vi "CabecalhoValvulaUnitariaV1.vi"(0 "Output File":path, 1 "Delta t":dbl=1.0, 2 "DAQ Rate":i32=5, 3 "SP CAME Frequency":dbl) -> (4 "data file":string="Data File:    created on Friday, December 03, 1999  at  4:41:37 PM\n\nWARNING: No tampering with this data please.\n\nTomasz W. Wysokinski   Cryofuel Systems Group © 1997/99.\n\n\n Abs. Time \t Run Time\tHCL-VLT\t HeatPipe \t GM-1 \tunused\t SHLD-1\t GM-2\t HCL-bottom\t M-1\t M-2\t SHLD-2\t Hall-P\t Magnet\r")   [LabVIEW 2019]
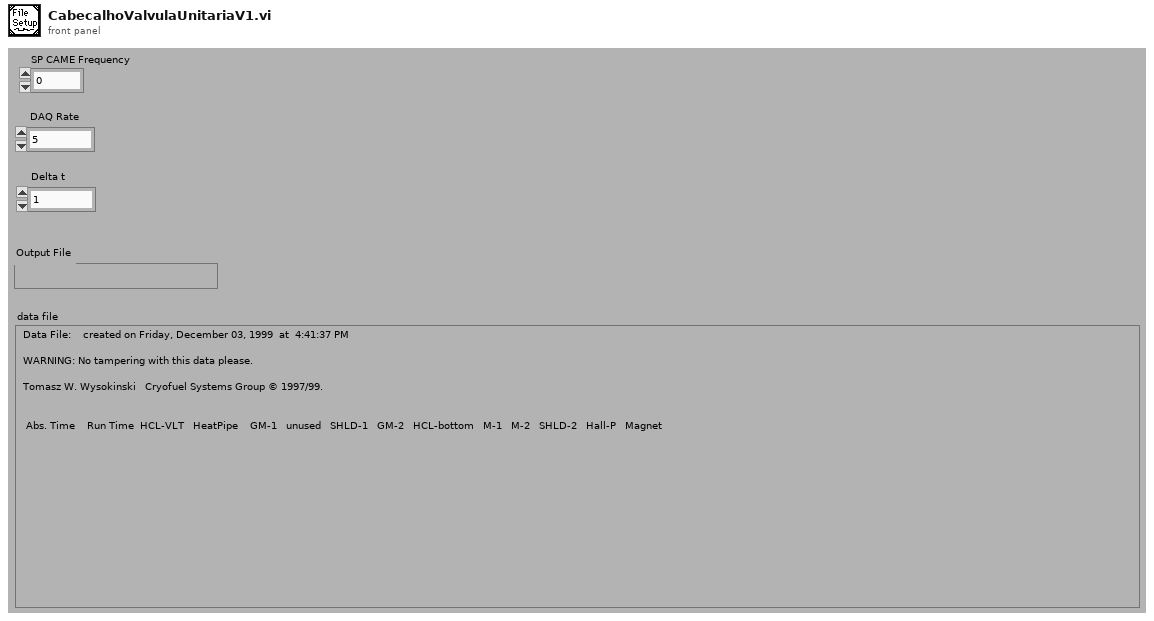
[diagram p1: front panel]
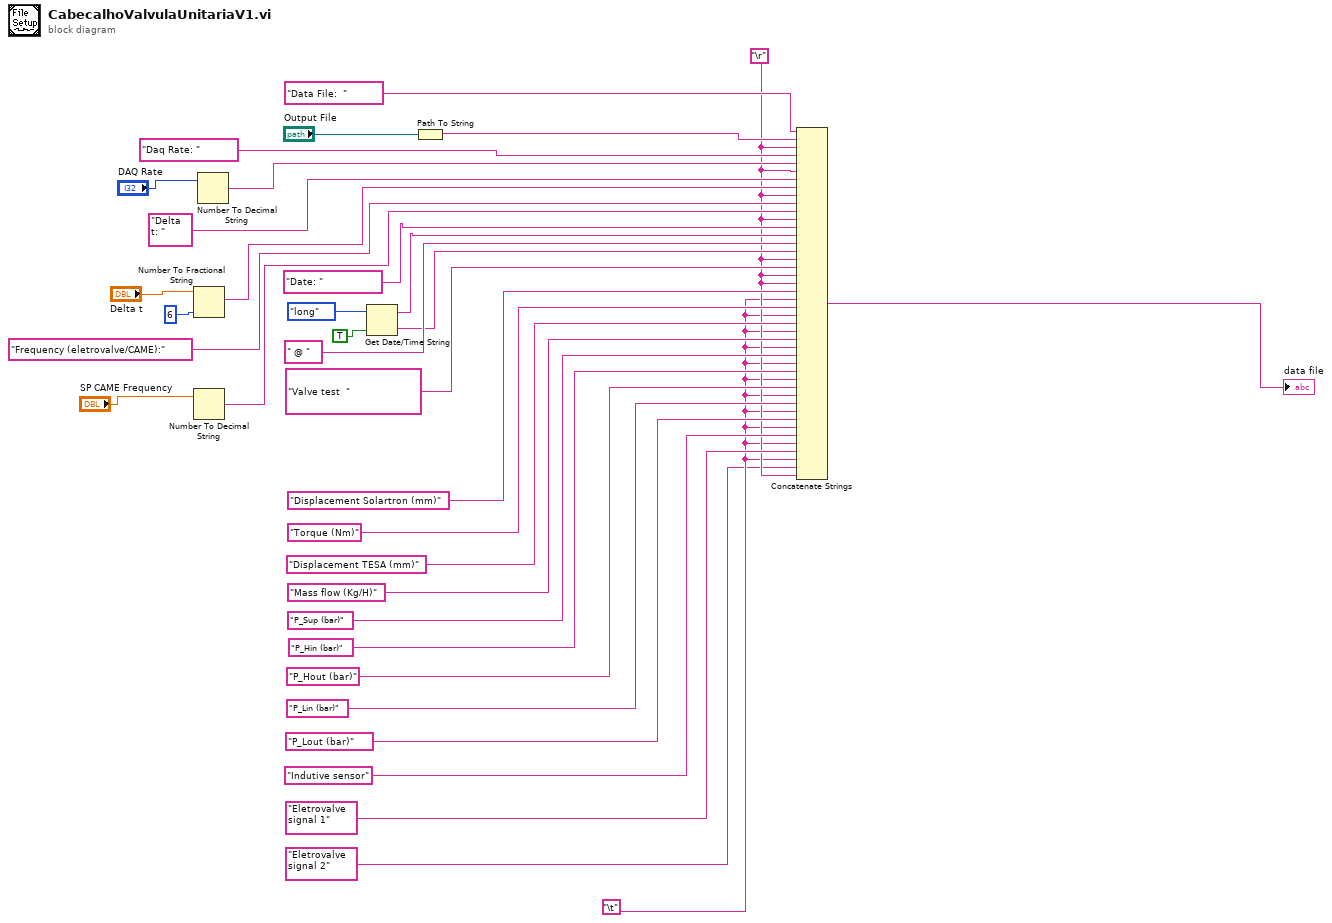
[diagram p0: block diagram]
diagram:
  w2 = "\t" ("time string")
  w3 = "\r"
  n1 = Number To Fractional String(number="Delta t", precision (6)=i16 6 ("width (-)")) -> (F-format string=w19:string)  [unwired: 2 in]
  n2 = Number To Decimal String(number="SP CAME Frequency") -> (decimal integer string=w10:string)  [unwired: 1 in]
  n3 = Number To Decimal String(number="DAQ Rate") -> (decimal integer string=w13:string)  [unwired: 1 in]
  n4 = Get Date/Time String(date format (0)=enum16{"short", "long", "abbreviated"}."long", want seconds? (F)=TRUE) -> (date string=w25:string, time string=w23:string)  [unwired: 1 out]
  n5 = Path To String(path="Output File") -> (string=w15:string)
  n6 = Concatenate Strings("Data File:  ", w15, w3, "Daq Rate: ", w13, w3, "Delta t: ", w19, w3, "Frequency (eletrovalve/CAME):", w10, w3, "Date: ", w25, " @ ", w23, w3, "Valve test  ", w3, w3, "Displacement Solartron (mm)", w2, "Torque (Nm)", w2, "Displacement TESA (mm)", w2, "Mass flow (Kg/H)", w2, "P_Sup (bar)", w2, "P_Hin (bar)", w2, "P_Hout (bar)", w2, "P_Lin (bar)", w2, "P_Lout (bar)", w2, "Indutive sensor", w2, "Eletrovalve signal 1", w2, "Eletrovalve signal 2", w3) -> (→"data file":string)
